vi "Longlasting one-axis command.vi"(0 "System no.":i32=1 min=1 max=4 step=1, 2 "Axis to command":string="A", 3 "Command":string="ATZ", 4 "Value":dbl=nan format="%.6f", 5 "error in":errorcluster, 6 "Axis and value?":bool, 12 "Stop refnum":refnum<vi>) -> (14 "Answer":bool, 15 "Stopped":bool, 19 "error out":errorcluster)   [LabVIEW 2026]
doc: "This VI sends a command (like REF, MNL or MPL), polls with #7 for controller-ready signal and returns original (boolean) command response."
panel:
  in  "Local stop":bool
  # "This vi sends a command (like REF, MNL or MPL), \npolls with #7 for controller ready signal and\nreturns original (boolean) command response."
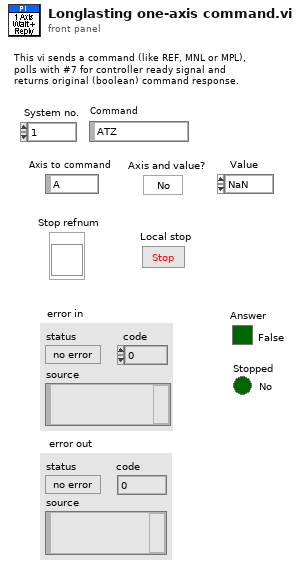
[diagram p1: front panel]
types:
  T1 = typedef "Semaphore RefNum" = refnum<k1>
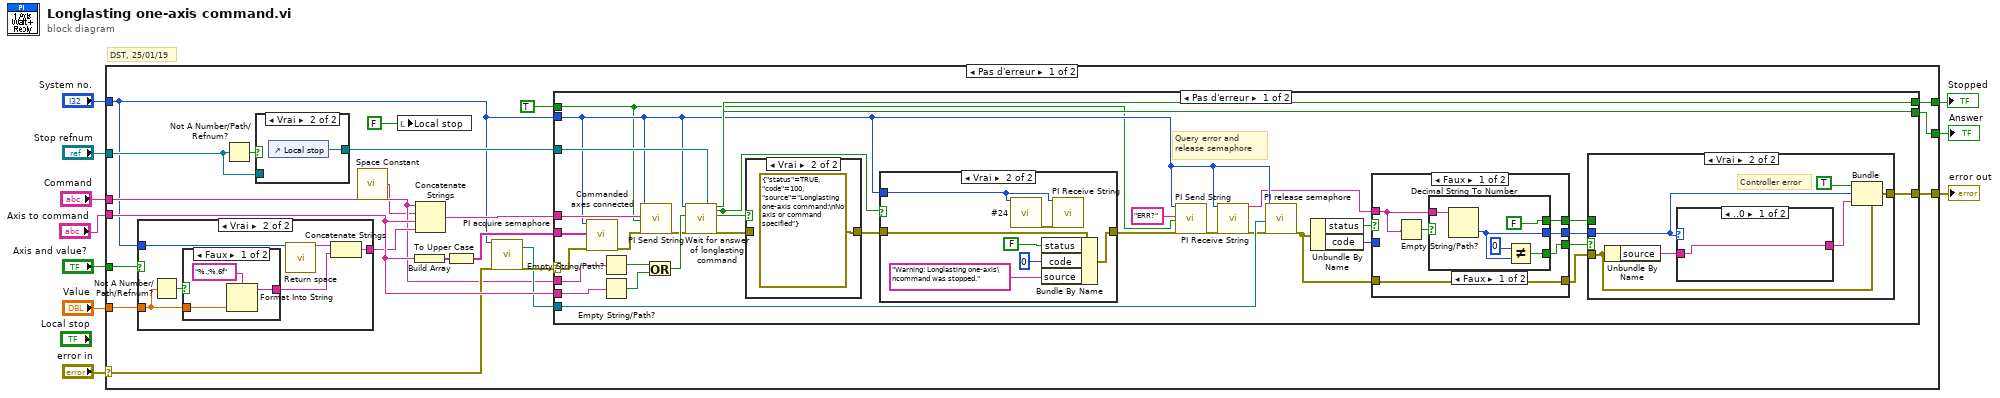
[diagram p0: block diagram]
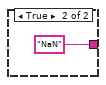
[diagram p4: hidden frame]
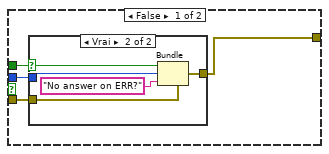
[diagram p6: hidden frame]
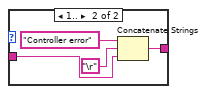
[diagram p8: hidden frame]
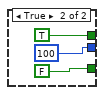
[diagram p9: hidden frame]
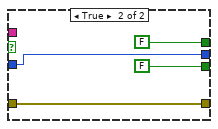
[diagram p10: hidden frame]
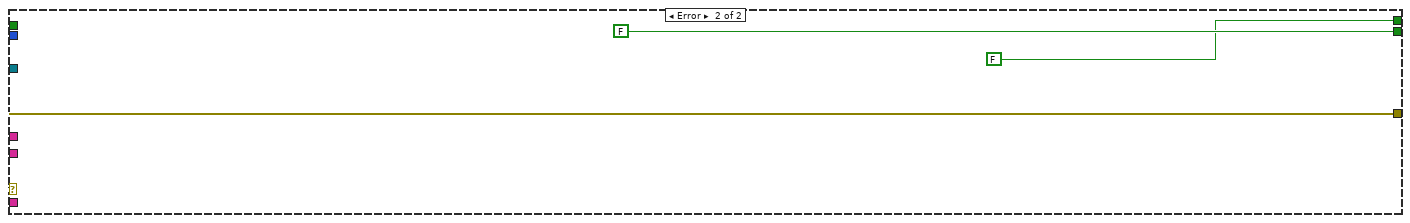
[diagram p12: hidden frame]
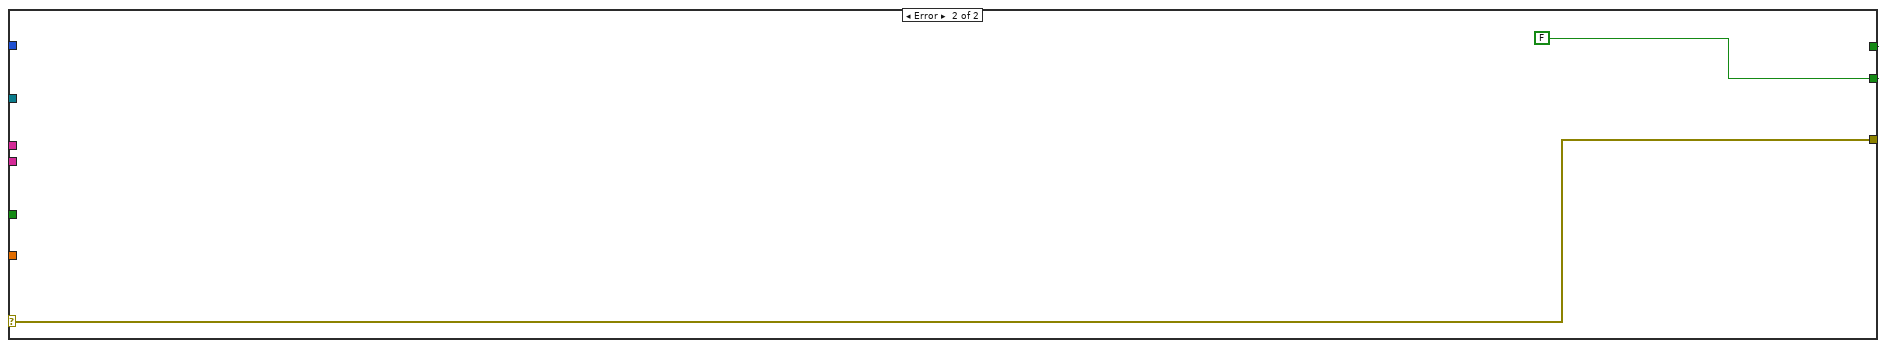
[diagram p13: hidden frame]
diagram:
  # "DST, 25/01/19"
  n1 = case shown="Pas d'erreur" "error in" {
    selector: "error in" -> [w18 w129]
    tunnel: "Axis to command" -> [w28 _]
    tunnel: [w27 w128] -> w9
    tunnel: "Axis and value?" -> [w26 _]
    tunnel: [w24 w129] -> w7
    tunnel: "System no." -> [w11 _]
    tunnel: "Value" -> [w17 _]
    tunnel: "Stop refnum" -> [w16 _]
    tunnel: "Command" -> [w15 _]
    tunnel: [w13 w128] -> w1
    frame No Error {
      n2 = case shown="Vrai" w26 {
        tunnel: ["" w36] -> w25
        tunnel: w11 -> [_ w38]
        tunnel: w17 -> [_ w35]
        frame False {
        }
        frame True {
          n3 = Not A Number/Path/Refnum?(number/path/refnum=w35) -> (NaN/Path/Refnum?=w40:bool)
          n4 = case shown="Faux" w40 {
            tunnel: w35 -> [w42 _]
            tunnel: [w41 "NaN"] -> w39
            frame False {
              n5 = Format Into String(format string="%.;%.6f" ("Format String"), w42) -> (resulting string=w41:string)  [unwired: 2 in, 1 out]
            }
            frame True {
            }
          }
          n6 = call "Return space.vi"("System no."=w38) -> ("String out"=w37:string)  [unwired: 1 in, 17 out]
          n7 = Concatenate Strings(w37, w39) -> (w36:string)
        }
      }
      n8 = Not A Number/Path/Refnum?(number/path/refnum=w16) -> (NaN/Path/Refnum?=w22:bool)
      n9 = case shown="Vrai" w22 {
        tunnel: [w32 w33] -> w21
        tunnel: w16 -> [w32 _]
        frame False {
        }
        frame True {
          n10 = control-ref of="Local stop"() -> (w33:refnum<vi>)
        }
      }
      n11 = call <vilib>:"Space Constant.vi"() -> ("String"=w14:string)
      n12 = local write "Local stop"(FALSE ("Stop loop")) -> ()
      n13 = Build Array(w28) -> (w30:string[])
      n14 = Concatenate Strings(w15, w14, w28, w25) -> (w31:string)
      n15 = To Upper Case(1:w30) -> (0:w29:string[])
      n16 = call "PI acquire semaphore.vi"("System no."=w11, "error in"=w18) -> ("semaphore out"=w19:T1, "error out"=w20:errorcluster)  [unwired: 16 out]
      n17 = case shown="Pas d'erreur" w20 {
        selector: w20 -> [w66 w126]
        tunnel: w31 -> [w75 _]
        tunnel: [w64 w126] -> w24
        tunnel: w29 -> [w73 _]
        tunnel: w11 -> [w62 _]
        tunnel: w28 -> [w59 _]
        tunnel: w15 -> [w61 _]
        tunnel: [w69 FALSE] -> w27
        tunnel: w21 -> [w68 _]
        tunnel: w19 -> [w63 _]
        tunnel: [w46 FALSE ("Stopped")] -> w13
        tunnel: TRUE ("Attach Linefeed?") -> [w45 _]
        frame No Error {
          # "Query error and\nrelease semaphore"
          n18 = call "Commanded axes connected.vi"("System no."=w62, "Commanded axes"=w73, "error in"=w66) -> ("error out"=w74:errorcluster)  [unwired: 1 in, 15 out]
          n19 = Empty String/Path?(string/path=w61) -> (empty?=w60:bool)
          n20 = Empty String/Path?(string/path=w59) -> (empty?=w58:bool)
          n21 = call "PI Send String.vi"("System no."=w62, "String to send"=w75, "Attach termination char.?"=w45, "error in"=w74) -> ("error out"=w71:errorcluster)  [unwired: 15 out]
          n22 = Or(x=w60, y=w58) -> (x .or. y?=w72:bool)
          n23 = call "Wait for answer of longlasting command.vi"("System no."=w62, "error in"=w71, "Stop refnum"=w68) -> ("Answer"=w69:bool, "Stopped"=w46:bool, "error out"=w70:errorcluster)  [unwired: 14 out]
          n24 = case shown="Vrai" w72 {
            tunnel: [w123 errorcluster {"status"=TRUE, "code"=100, "source"="Longlasting one-axis command:\nNo axis or command specified"} ("error out")] -> w67
            tunnel: w70 -> [w123 _]
            frame False {
            }
            frame True {
            }
          }
          n25 = case shown="Vrai" w46 {
            tunnel: w62 -> [_ w83]
            tunnel: w67 -> [w76 w77]
            tunnel: [w76 w78] -> w65
            frame False {
            }
            frame True {
              n26 = call "#24.vi"("System no."=w83) -> ("error out"=w82:errorcluster)  [unwired: 1 in, 17 out]
              n27 = Bundle By Name(cluster=w77, "status"=FALSE, "code"=0, "source"="Warning: Longlasting one-axis\ncommand was stopped.") -> (w78:errorcluster)
              n28 = call "PI Receive String.vi"("System no."=w83, "error in"=w82) -> ()  [unwired: 1 in, 17 out]
            }
          }
          n29 = call "PI Send String.vi"("System no."=w62, "String to send"="ERR?", "Attach termination char.?"=w45, "error in"=w65) -> ("error out"=w55:errorcluster)  [unwired: 15 out]
          n30 = call "PI Receive String.vi"("System no."=w62, "error in"=w55) -> ("String read"=w53:string, "error out"=w52:errorcluster)  [unwired: 1 in, 15 out]
          n31 = call "PI release semaphore.vi"("System no."=w62, "semaphore"=w63, "error in"=w52) -> ("error out"=w48:errorcluster)  [unwired: 1 in, 15 out]
          n32 = Unbundle By Name(w48) -> ("status"=w49:bool, "code"=w50:i32)
          n33 = case shown="Faux" w49 {
            tunnel: w53 -> [w106 _]
            tunnel: [w110 FALSE ("Controller Error")] -> w51
            tunnel: [w109 w121] -> w57
            tunnel: w50 -> [_ w121]
            tunnel: [w108 FALSE ("Controller Error")] -> w56
            tunnel: [w105 w119] -> w47
            tunnel: w48 -> [w105 w119]
            frame False {
              n34 = Empty String/Path?(string/path=w106) -> (empty?=w107:bool)
              n35 = case shown="Faux" w107 {
                tunnel: [w115 FALSE] -> w110
                tunnel: w106 -> [w113 _]
                tunnel: [w112 100] -> w109
                tunnel: [FALSE TRUE] -> w108
                frame False {
                  n36 = Decimal String To Number(string=w113) -> (number=w112:i32)  [unwired: 3 out]
                  n37 = Not Equal?(x=0, y=w112) -> (x != y?=w115:bool)
                }
                frame True {
                }
              }
            }
            frame True {
            }
          }
          n38 = case shown="Vrai" w51 {
            tunnel: w57 -> [w84 w97]
            tunnel: [w86 w99] -> w64
            tunnel: w47 -> [w87 w94]
            tunnel: w56 -> [w85 _]
            frame False {
              n39 = case shown="Vrai" w85 {
                selector: w85 -> [_ w90]
                tunnel: w87 -> [w88 w89]
                tunnel: [w88 w91] -> w86
                tunnel: w84 -> [_ w93]
                frame False {
                }
                frame True {
                  n40 = Bundle(cluster=w89, "status"=w90, "code"=w93, "source"="No answer on ERR?") -> (w91:errorcluster)
                }
              }
            }
            frame True {
              # "Controller error"
              n41 = Unbundle By Name(w94) -> ("source"=w95:string)
              n42 = case shown="..0" w97 {
                tunnel: [w100 w104] -> w96
                tunnel: w95 -> [w100 w101]
                frame ..0 {
                }
                frame 1.. {
                  n43 = Concatenate Strings("Controller error", "\r" ("Substring"), w101) -> (w104:string)
                }
              }
              n44 = Bundle(cluster=w94, "status"=TRUE, "code"=w97, "source"=w96) -> (w99:errorcluster)
            }
          }
        }
        frame Error {
        }
      }
    }
    frame Error {
      w128 = FALSE ("Answer")
    }
  }
  "error out" <- w7
  "Answer" <- w9
  "Stopped" <- w1
